vi "CRYGet Table Click State.vi"(10 "Coords":T1, 11 "Table Ref In":refnum<vi>) -> (0 "Column":i32, 1 "Row":i32, 2 "State":bool, 3 "Table Ref Out":refnum<vi>)   [LabVIEW 2013]
uses:
  <vilib>/Utility/miscctls.llb/LVPoint32TypeDef.ctl
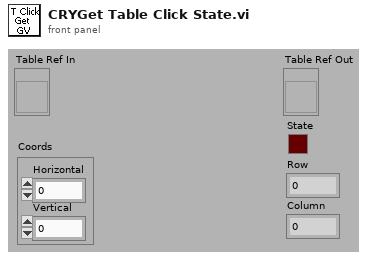
[diagram p1: front panel]
types:
  T1 = typedef "LVPoint32TypeDef.ctl" = cluster{"Horizontal":i32, "Vertical":i32}
  T2 = typedef "LVRowAndColumnTypeDef.ctl" = cluster{"Row":i32, "Column":i32}
  T3 = typedef "LVBoundsTypeDef.ctl" = cluster{"Width":u32, "Height":u32}
  T4 = typedef "LVPositionTypeDef.ctl" = cluster{"Left":i32, "Top":i32}
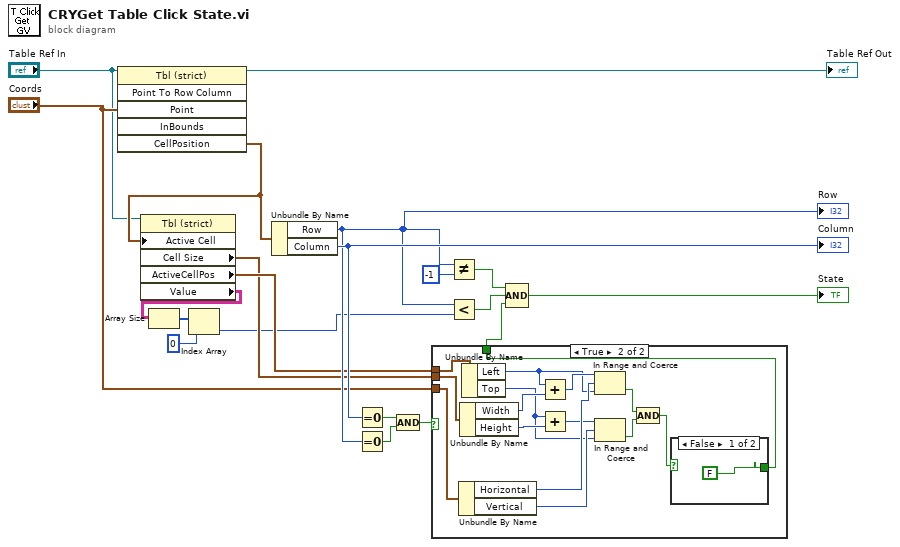
[diagram p0: block diagram]
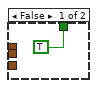
[diagram p2: hidden frame]
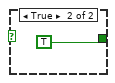
[diagram p3: hidden frame]
diagram:
  n1 = invoke class="Tbl (strict)" method="Point To Row Column"(reference="Table Ref In", "Point"="Coords") -> (reference out=→"Table Ref Out":refnum<vi>, "CellPosition"=w6:T2)  [unwired: 4 in, 4 out]
  n2 = property on="Property Node" class="Tbl (strict)"(reference="Table Ref In", "Active Cell"=w6) -> ("Cell Size"=w7:T3, "ActiveCellPos"=w8:T4, "Value"=w5:string[][])  [unwired: 1 in, 2 out]
  n3 = Array Size(array=w5) -> (size(s)=w4:i32[])
  n4 = Index Array(array=w4, index=0) -> (element=w1:i32)
  n5 = Unbundle By Name(w6) -> ("Row"=w12:i32, "Column"=w13:i32)
  "Row" <- w12
  "Column" <- w13
  n6 = Equal To 0?(x=w13) -> (x = 0?=w17:bool)
  n7 = Equal To 0?(x=w12) -> (x = 0?=w16:bool)
  n8 = Compound Arithmetic op=AND(w17, w16) -> (w15:bool)
  n9 = case shown="True" w15 {
    tunnel: w8 -> [_ w35]
    tunnel: "Coords" -> [_ w36]
    tunnel: w7 -> [_ w34]
    tunnel: [TRUE w22] -> w14
    frame False {
    }
    frame True {
      n10 = Unbundle By Name(w36) -> ("Horizontal"=w27:i32, "Vertical"=w31:i32)
      n11 = Unbundle By Name(w34) -> ("Width"=w33:u32, "Height"=w32:u32)
      n12 = Unbundle By Name(w35) -> ("Left"=w25:i32, "Top"=w23:i32)
      n13 = Add(x=w25, y=w33) -> (x+y=w26:u32)
      n14 = Add(x=w23, y=w32) -> (x+y=w24:u32)
      n15 = In Range and Coerce(upper limit=w26, x=w27, lower limit=w25) -> (In Range?=w30:bool)  [unwired: 1 out]
      n16 = In Range and Coerce(upper limit=w24, x=w31, lower limit=w23) -> (In Range?=w29:bool)  [unwired: 1 out]
      n17 = Compound Arithmetic op=AND(w30, w29) -> (w28:bool)
      n18 = case shown="False" w28 {
        tunnel: [FALSE TRUE] -> w22
        frame False {
        }
        frame True {
        }
      }
    }
  }
  n19 = Not Equal?(x=w12, y=-1) -> (x != y?=w18:bool)
  n20 = Less?(x=w12, y=w1) -> (x < y?=w19:bool)
  n21 = Compound Arithmetic op=AND(w18, w19, w14) -> (→"State":bool)
